vi "Test Positive Definite.vi"   [LabVIEW 2018, in "NI_AALPro.lvlib"]
doc: "Tests whether <B>Input Matrix</B> is a complex-conjugate symmetric and positive definite matrix. The data type you wire to the <B>Input Matrix</B> input determines the polymorphic instance to use."
uses:
  NI_AALPro.lvlib
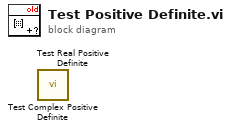
[diagram p0: block diagram]
diagram:
  n1 = call "Test Complex Positive Definite.vi"() -> ()  [unwired: 1 in, 2 out]
  n2 = call "Test Real Positive Definite.vi"() -> ()  [unwired: 1 in, 2 out]
